vi "RegisterVIs.vi"(8 "error in":errorcluster, 10 "VI References":refnum<vi>[](array[refnum])) -> (0 "error out":errorcluster, 1 "Current Language":string)   [LabVIEW 2020]
doc: "Register VI(s) to the localizer's registry. Automatically applies the current language to these VIs."
uses:
  Localization FGV Action -- Enum.ctl
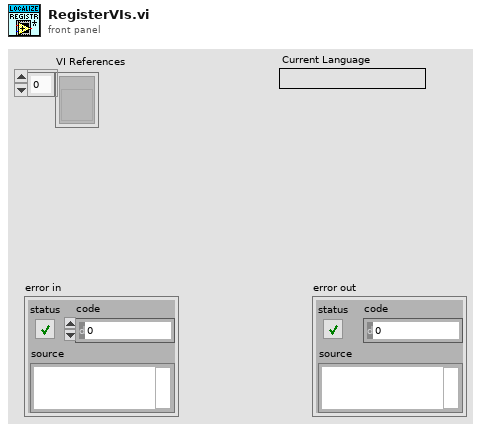
[diagram p1: front panel]
types:
  T1 = typedef "Localization FGV Action -- Enum.ctl" = enum16{"Read Dictionary", "Translate VIs", "Register VI", "Get Languages", "Translate Phrase", "Get Key For Phrase", "Get Phrase For Phrase", "Translate VI", "Unregister"}
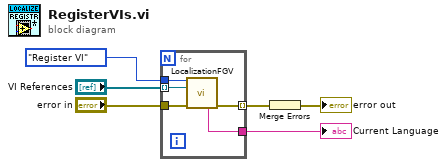
[diagram p0: block diagram]
diagram:
  n1 = for {
    tunnel: Localization_FGV_Action_--_Enum."Register VI" ("Action") -> [w11]
    tunnel: "error in" -> [w10]
    tunnel: [w9] -> w4 mode=indexing
    tunnel: "VI References" -> [w8] mode=indexing
    tunnel: [w7] -> w1
    n2 = call "LocalizationFGV.vi"("Action"=w11, "VI in"=w8, "error in"=w10) -> ("Current Language"=w7:string, "error out"=w9:errorcluster)  [unwired: 7 in, 4 out]
  }
  "Current Language" <- w1
  n3 = Merge Errors(w4) -> (→"error out":errorcluster)
